vi "SCOPE_OPEN.vi"(8 "error in (no error)":errorcluster, 9 "Clear Error w/ Report?":bool, 10 "Configuration Cluster":T1={"General"={"Config.ini"=path "", "Default Logging Path"=path ""}, "Hardware"={"Global T VAR"="", "Global B VAR"="", "VISAS"={"GEN COM"="", "SCOPE COM"="", "VNA COM"=""}}, "Operation"={"Operation Mode"=enum."Idle-Off", "Status"="", "NewLog?"=FALSE, "OvenWarn"=FALSE, "Scope Settings"={"TimeBase"=0.0, "VerticalScale"=4.0}}}) -> (0 "error out":errorcluster, 1 "Success?":bool, 2 "Configuration Cluster Out":T1={"General"={"Config.ini"=path "", "Default Logging Path"=path ""}, "Hardware"={"Global T VAR"="", "Global B VAR"="", "VISAS"={"GEN COM"="", "SCOPE COM"="", "VNA COM"=""}}, "Operation"={"Operation Mode"=enum."Idle-Off", "Status"="", "NewLog?"=FALSE, "OvenWarn"=FALSE, "Scope Settings"={"TimeBase"=0.0, "VerticalScale"=4.0}}}, 4 "message":string)   [LabVIEW 2021]
uses:
  Config_Cluster.ctl
  Mode_Enum.ctl
  <vilib>/Utility/error.llb/DialogType.ctl
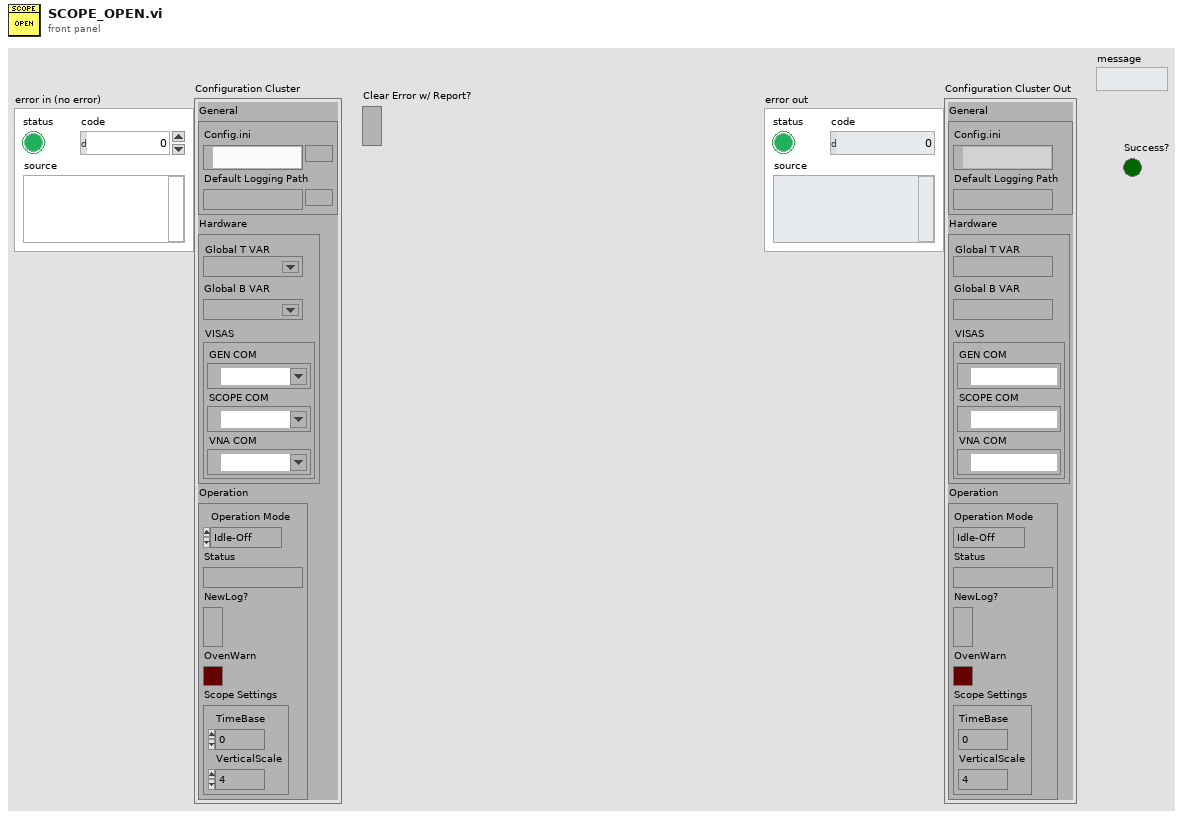
[diagram p1: front panel]
types:
  T1 = typedef "Config_Cluster.ctl" = cluster{"General":cluster{"Config.ini":path, "Default Logging Path":path}, "Hardware":cluster{"Global T VAR":refnum<k21>, "Global B VAR":refnum<k21>, "VISAS":cluster{"GEN COM":refnum<visa-resource-name>, "SCOPE COM":refnum<visa-resource-name>, "VNA COM":refnum<visa-resource-name>}}, "Operation":cluster{"Operation Mode":T2, "Status":string, "NewLog?":bool, "OvenWarn":bool, "Scope Settings":cluster{"TimeBase":dbl, "VerticalScale":dbl}}}
  T2 = typedef "Mode_Enum.ctl" = enum16{"OvenNRDY", "Logging", "Idle-Off", "Idle"}
  T3 = typedef "DialogType.ctl" = u16
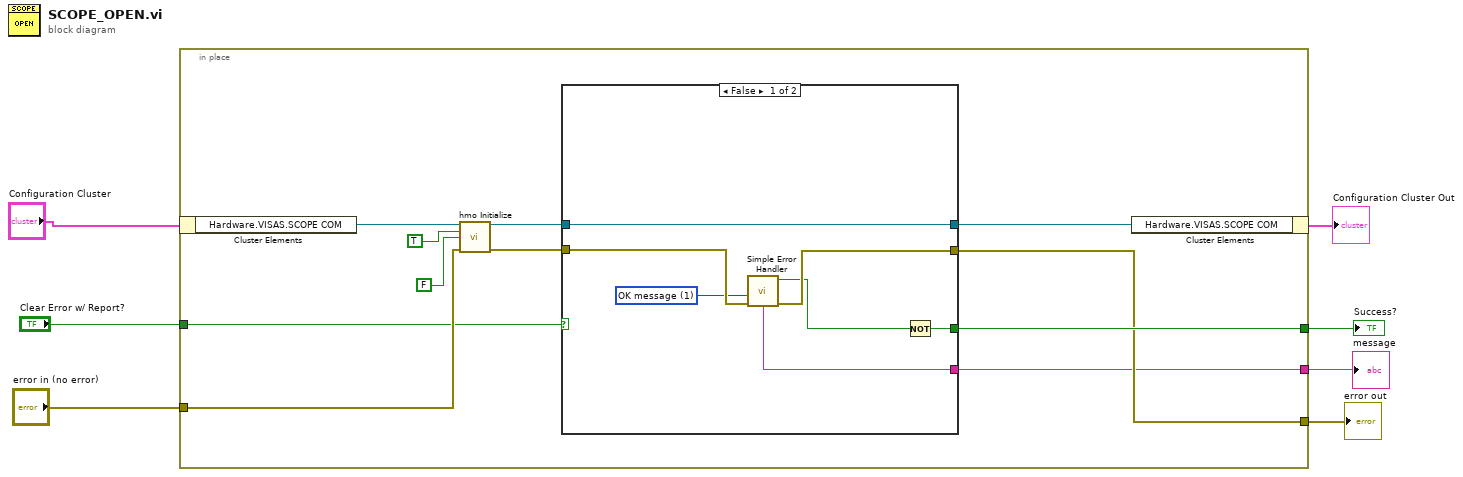
[diagram p0: block diagram]
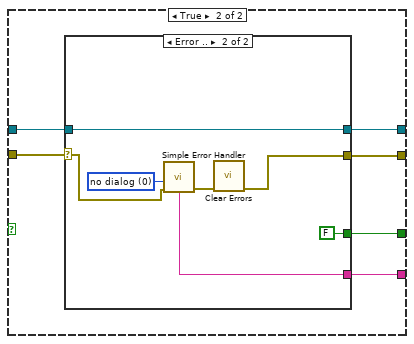
[diagram p2: hidden frame]
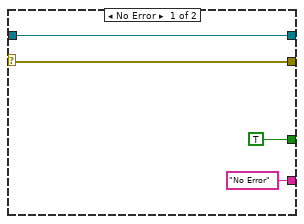
[diagram p3: hidden frame]
diagram:
  n1 = in-place {
    in-place-border: "error in (no error)" -> [w17]
    in-place-border: [w9] -> w4
    in-place-border: "Clear Error w/ Report?" -> [w14]
    in-place-border: [w11] -> w2
    in-place-border: [w8] -> w1
    n2 = in-place-cluster #1("Configuration Cluster") -> ("Hardware.VISAS.SCOPE COM"=w18:refnum<visa-resource-name>)
    n3 = call <instrlib>:"hmo Initialize.vi"("VISA resource name"=w18, "ID Query (T: Check)"=TRUE, "Reset (T: Reset)"=FALSE, "error in (no error)"=w17) -> ("VISA resource name out"=w12:refnum<visa-resource-name>, "error out"=w13:errorcluster)  [unwired: 10 in]
    n4 = case shown="False" w14 {
      tunnel: w13 -> [w24 w31]
      tunnel: w12 -> [w25 w30]
      tunnel: [w22 w29] -> w11
      tunnel: [w25 w28] -> w10
      tunnel: [w23 w27] -> w9
      tunnel: [w19 w26] -> w8
      frame False {
        w20 = T3 1 items=["no dialog", "OK message", "continue or stop message", "OK message + warnings", "continue/stop + warnings"] ("type of dialog (OK msg:1)")
        n5 = call <vilib>:"Simple Error Handler.vi"("type of dialog (OK msg:1)"=w20, "error in (no error)"=w24) -> ("error?"=w21:bool, "error out"=w23:errorcluster, "message"=w19:string)  [unwired: 3 in, 2 out]
        n6 = Not(x=w21) -> (.not. x?=w22:bool)
      }
      frame True {
        n7 = case shown="Error .." w31 {
          selector: w31 -> [w33 w39]
          tunnel: w30 -> [w34 w41]
          tunnel: [TRUE FALSE] -> w29
          tunnel: [w34 w41] -> w28
          tunnel: [w33 w37] -> w27
          tunnel: ["No Error" ("message") w36] -> w26
          frame No Error {
          }
          frame Error {
            w40 = T3 0 items=["no dialog", "OK message", "continue or stop message", "OK message + warnings", "continue/stop + warnings"] ("type of dialog (OK msg:1)")
            n8 = call <vilib>:"Simple Error Handler.vi"("type of dialog (OK msg:1)"=w40, "error in (no error)"=w39) -> ("error out"=w38:errorcluster, "message"=w36:string)  [unwired: 3 in, 3 out]
            n9 = call <vilib>:"Clear Errors.vi"("error in (no error)"=w38) -> ("error out"=w37:errorcluster)  [unwired: 5 in, 1 out]
          }
        }
      }
    }
    n10 = in-place-cluster #1("Hardware.VISAS.SCOPE COM"=w10) -> (→"Configuration Cluster Out":T1)
  }
  "error out" <- w4
  "Success?" <- w2
  "message" <- w1
